vi "SetIntensityBounds.vi"(0 "upper_bound":dbl format="%#_13g", 1 "lower_bound":dbl format="%#_13g", 3 "whichGraph":i32, 4 "LabVIEW Web Service Request":refnum<class "Web Request.lvclass">) -> ()   [LabVIEW 2016]
uses:
  <vilib>/wsapi/Web Request.lvclass
  <vilib>/wsapi/NI_WebServices.lvlib
panel:
  in  "Transconductance.. 2":refnum<vi>
  out "error out":errorcluster
  in  "error in (no error)":errorcluster
  out "Intensity Graph":dbl[][](graph)
  # "Use the Web Service Request input terminal to call the VIs on the Web Services palette. Do not remove it from the connector pane unless you don't need access to the palette."
  # "Each additional control wired to the connector pane will be available as an input in the URL. To include an indicator in terminal-mode output (the default setting), it must also be wired to the connector pane."
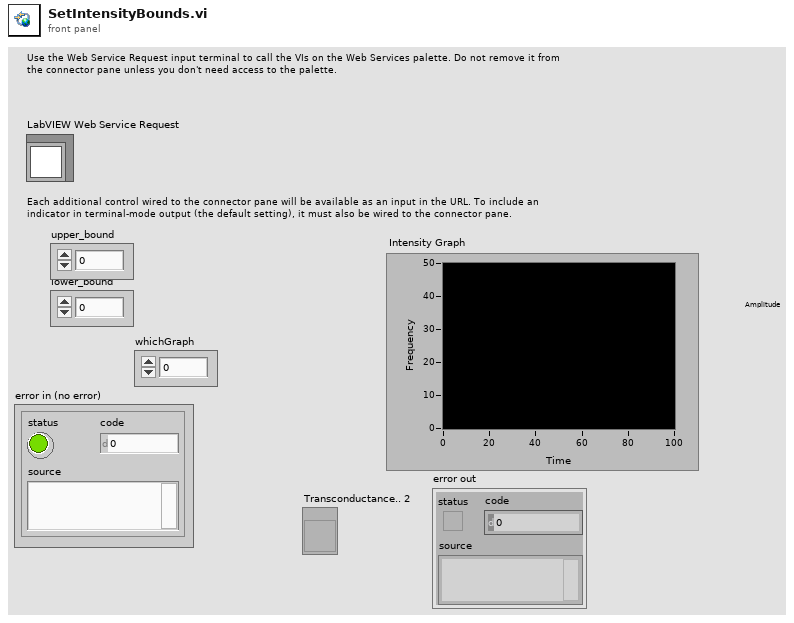
[diagram p1: front panel]
types:
  T1 = typedef "imagedata.ctl" = cluster{"image type":i32, "image depth":i32, "image":u8[], "mask":u8[], "colors":u32[], "Rectangle":cluster{"left":i16, "top":i16, "right":i16, "bottom":i16}}
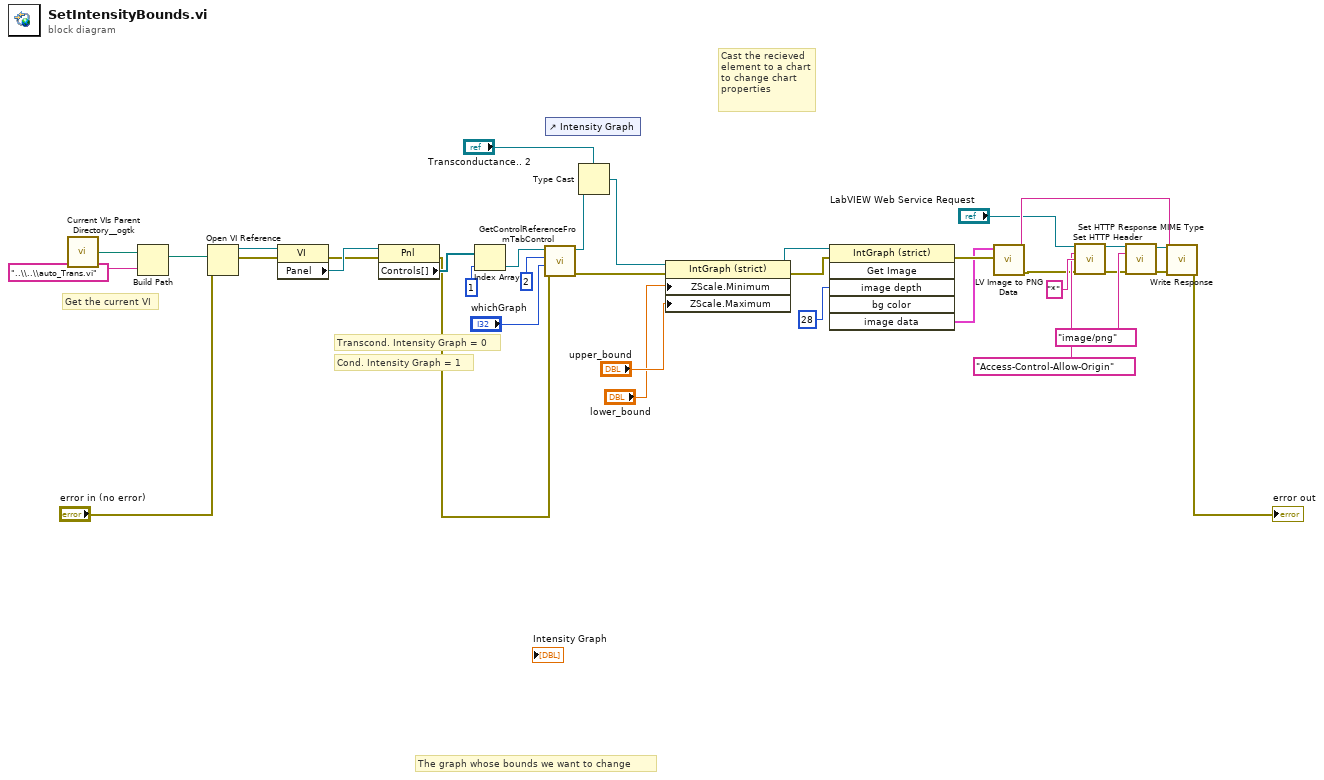
[diagram p0: block diagram]
diagram:
  # "Cond. Intensity Graph = 1"
  # "Cast the recieved element to a chart to change chart properties"
  # "Transcond. Intensity Graph = 0"
  # "Get the current VI"
  # "The graph whose bounds we want to change"
  n1 = call <userlib>:"Current VIs Parent Directory__ogtk.vi"() -> ("Parent Directory (+ Relative)"=w33:path)  [unwired: 5 in]
  n2 = Build Path(base path=w33, name or relative path="..\\..\\auto_Trans.vi") -> (appended path=w31:path)
  n3 = Open VI Reference(vi path=w31, error in (no error)="error in (no error)") -> (vi reference=w34:refnum<vi>, error out=w22:errorcluster)  [unwired: 4 in]
  n4 = property class="VI"(reference=w34, error in=w22) -> (error out=w27:errorcluster, "Panel"=w30:refnum<vi>)  [unwired: 1 out]
  n5 = property class="Pnl"(reference=w30, error in=w27) -> (error out=w14:errorcluster, "Controls[]"=w29:refnum<vi>[])  [unwired: 1 out]
  n6 = Index Array(array=w29, index=1) -> (element=w28:refnum<vi>)
  n7 = call "GetControlReferenceFromTabControl.vi"("error in (no error)"=w14, "control"="whichGraph", "page"=2 ("index"), "Ctl Refnum"=w28) -> ("error out"=w17:errorcluster, "element"=w23:refnum<vi>)  [unwired: 6 in]
  n8 = control-ref of="Intensity Graph"() -> ()  [unwired: 1 out]
  n9 = Type Cast(type="Transconductance.. 2", x=w23) -> (*(type *) &x=w18:refnum<vi>)
  n10 = property class="IntGraph (strict)"(reference=w18, error in=w17, "ZScale.Minimum"="lower_bound", "ZScale.Maximum"="upper_bound") -> (reference out=w16:refnum<vi>, error out=w15:errorcluster)
  n11 = invoke class="IntGraph (strict)" method="Get Image"(reference=w16, error in=w15, "image depth"=28 ("Image Depth")) -> (error out=w26:errorcluster, "image data"=w25:T1)  [unwired: 3 in, 4 out]
  n12 = call <vilib>:"LV Image to PNG Data.vi"("error in (no error)"=w26, "image data"=w25) -> ("error out"=w1:errorcluster, "png data"=w35:string)  [unwired: 8 in]
  n13 = call <vilib>:"Set HTTP Header.vi"("LabVIEW Web Service Request"="LabVIEW Web Service Request", "header"="Access-Control-Allow-Origin", "header value"="*", "error in (no error)"=w1) -> ("LabVIEW Web Service Request out"=w7:refnum<class "Web Request.lvclass">, "error out"=w4:errorcluster)  [unwired: 10 in]
  n14 = call <vilib>:"Set HTTP Response MIME Type.vi"("LabVIEW Web Service Request"=w7, "MIME type (text/html)"="image/png", "error in (no error)"=w4) -> ("LabVIEW Web Service Request out"=w2:refnum<class "Web Request.lvclass">, "error out"=w3:errorcluster)  [unwired: 11 in]
  n15 = call <vilib>:"Write Response.vi"("LabVIEW Web Service Request"=w2, "response string"=w35, "error in (no error)"=w3) -> ("error out"=→"error out":errorcluster)  [unwired: 11 in, 1 out]
